vi "VCS Halt Velocity Movement.vi"(8 "error in (no error)":errorcluster, 11 "axis in":cluster{"keyHandle":u32, "nodeId":u16}={"keyHandle"=0, "nodeId"=1}) -> (0 "error out":errorcluster, 3 "axis out":cluster{"keyHandle":u32, "nodeId":u16}={"keyHandle"=0, "nodeId"=1})   [LabVIEW 2019, in "maxonEPOS.lvlib"]
doc: "With function <B>VCS Halt Velocity Movement</B> movement stops with profile deceleration."
uses:
  Examples/maxonEPOS.lvlib
  Resources/EposCmd.dll
  Resources/EposCmd64.dll
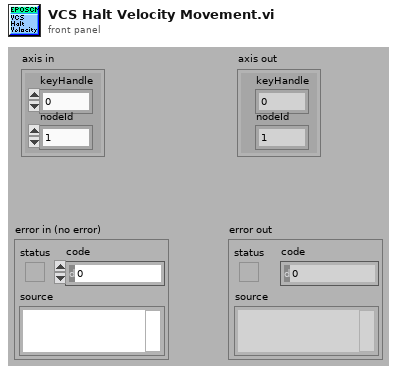
[diagram p1: front panel]
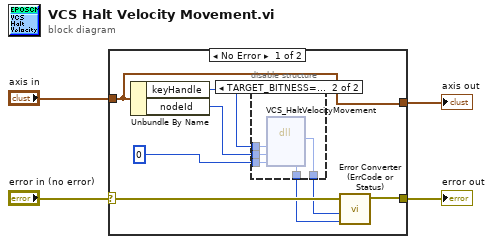
[diagram p0: block diagram]
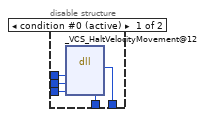
[diagram p2: hidden frame]
diagram:
  n1 = case shown="No Error" "error in (no error)" {
    selector: "error in (no error)" -> [w12 w24]
    tunnel: [w11 w24] -> w3
    tunnel: "axis in" -> [w7 w23]
    tunnel: [w7 w23] -> w1
    frame No Error {
      n2 = Unbundle By Name(w7) -> ("keyHandle"=w9:u32, "nodeId"=w8:u16)
      n3 = disable-structure shown="TARGET_BITNESS==64" {
        disable-tunnel: [w17 w22] -> w10
        disable-tunnel: w9 -> [w16 w21]
        disable-tunnel: w8 -> [w15 w20]
        disable-tunnel: u32 0 ("pErrorCode") -> [w14 w19]
        disable-tunnel: [w13 w18] -> w5
        frame condition #0 (active) {
          n4 = dll-call lib="C:/workspace/project/scancon/sw/SSI_Tool/InstrumentsInterfaces/Motordriver/maxon EPOS/Resources/EposCmd.*" fn="_VCS_HaltVelocityMovement@12"("KeyHandle"=w16, "NodeId"=w15, "pErrorCode"=w14) -> (w13:i32, "pErrorCode"=w17:u32)  [unwired: 5 in, 2 out]
        }
        frame condition #1 {
          n5 = dll-call lib="C:/Sources/LabView/maxon EPOS/Resources/EposCmd64.*" fn="VCS_HaltVelocityMovement" ("EposCmd.dll:_VCS_HaltVelocityMovement@12")("KeyHandle"=w21, "NodeId"=w20, "pErrorCode"=w19) -> ("Rückgabetyp"=w18:i32, "pErrorCode"=w22:u32)  [unwired: 5 in, 2 out]
        }
      }
      n6 = call "Error Converter (ErrCode or Status).vi"("error code"=w10, "return type"=w5, "error in (no error)"=w12) -> ("error out"=w11:errorcluster)  [unwired: 7 in]
    }
    frame Error {
    }
  }
  "error out" <- w3
  "axis out" <- w1
